vi "LiveAcquire Callback.vi"(4 "Config And DataQueues":T1 {"Config In"."Hardware Configuration"."Lasers Configuration"."SettingValues"."785 Power" format="%.1f"; "Config In"."Hardware Configuration"."Lasers Configuration"."SettingValues"."647 Power" format="%.1f"; "Config In"."Hardware Configuration"."Lasers Configuration"."SettingValues"."561 Power" format="%.1f"}, 5 "Event Data":cluster{"sender":refnum<k24>, "e":refnum<k24>}, 6 "Control Ref":refnum<k24>, 7 "Event Common Data":T10) -> ()   [LabVIEW 2019]
uses:
  C:/RM21-MMicrosopeSource/HardwareAdapter/Camera/Dependencies/PVCamNET.dll
  HardwareAdapter/Camera/Dependencies/PVCamNET.dll
  Config DataQueues And Notifier Ctl.ctl
  DataQueuesAndNotifier.ctl
  Settings/System Running Settings.ctl
  HardwareAdapter/Support/Hardware Configuration.ctl
  HardwareAdapter/Support/Camera Configuration.ctl
  <vilib>/vision/Image Controls.llb/IMAQ Image.ctl
  C:/RM21-MMicrosopeSource/HardwareAdapter/Lasers/Dependencies/Oxxius_Boxx.dll
  HardwareAdapter/Lasers/Dependencies/Oxxius_Boxx.dll
  Logging/Logging Configuration.ctl
  Controls/DeviceStatusCtl.ctl
  Controls/CallBack Refs.ctl
  Controls/Image MatadataCtl.ctl
  Global.vi
  Logging/Logging.lvlib
  Settings/Settings.lvlib
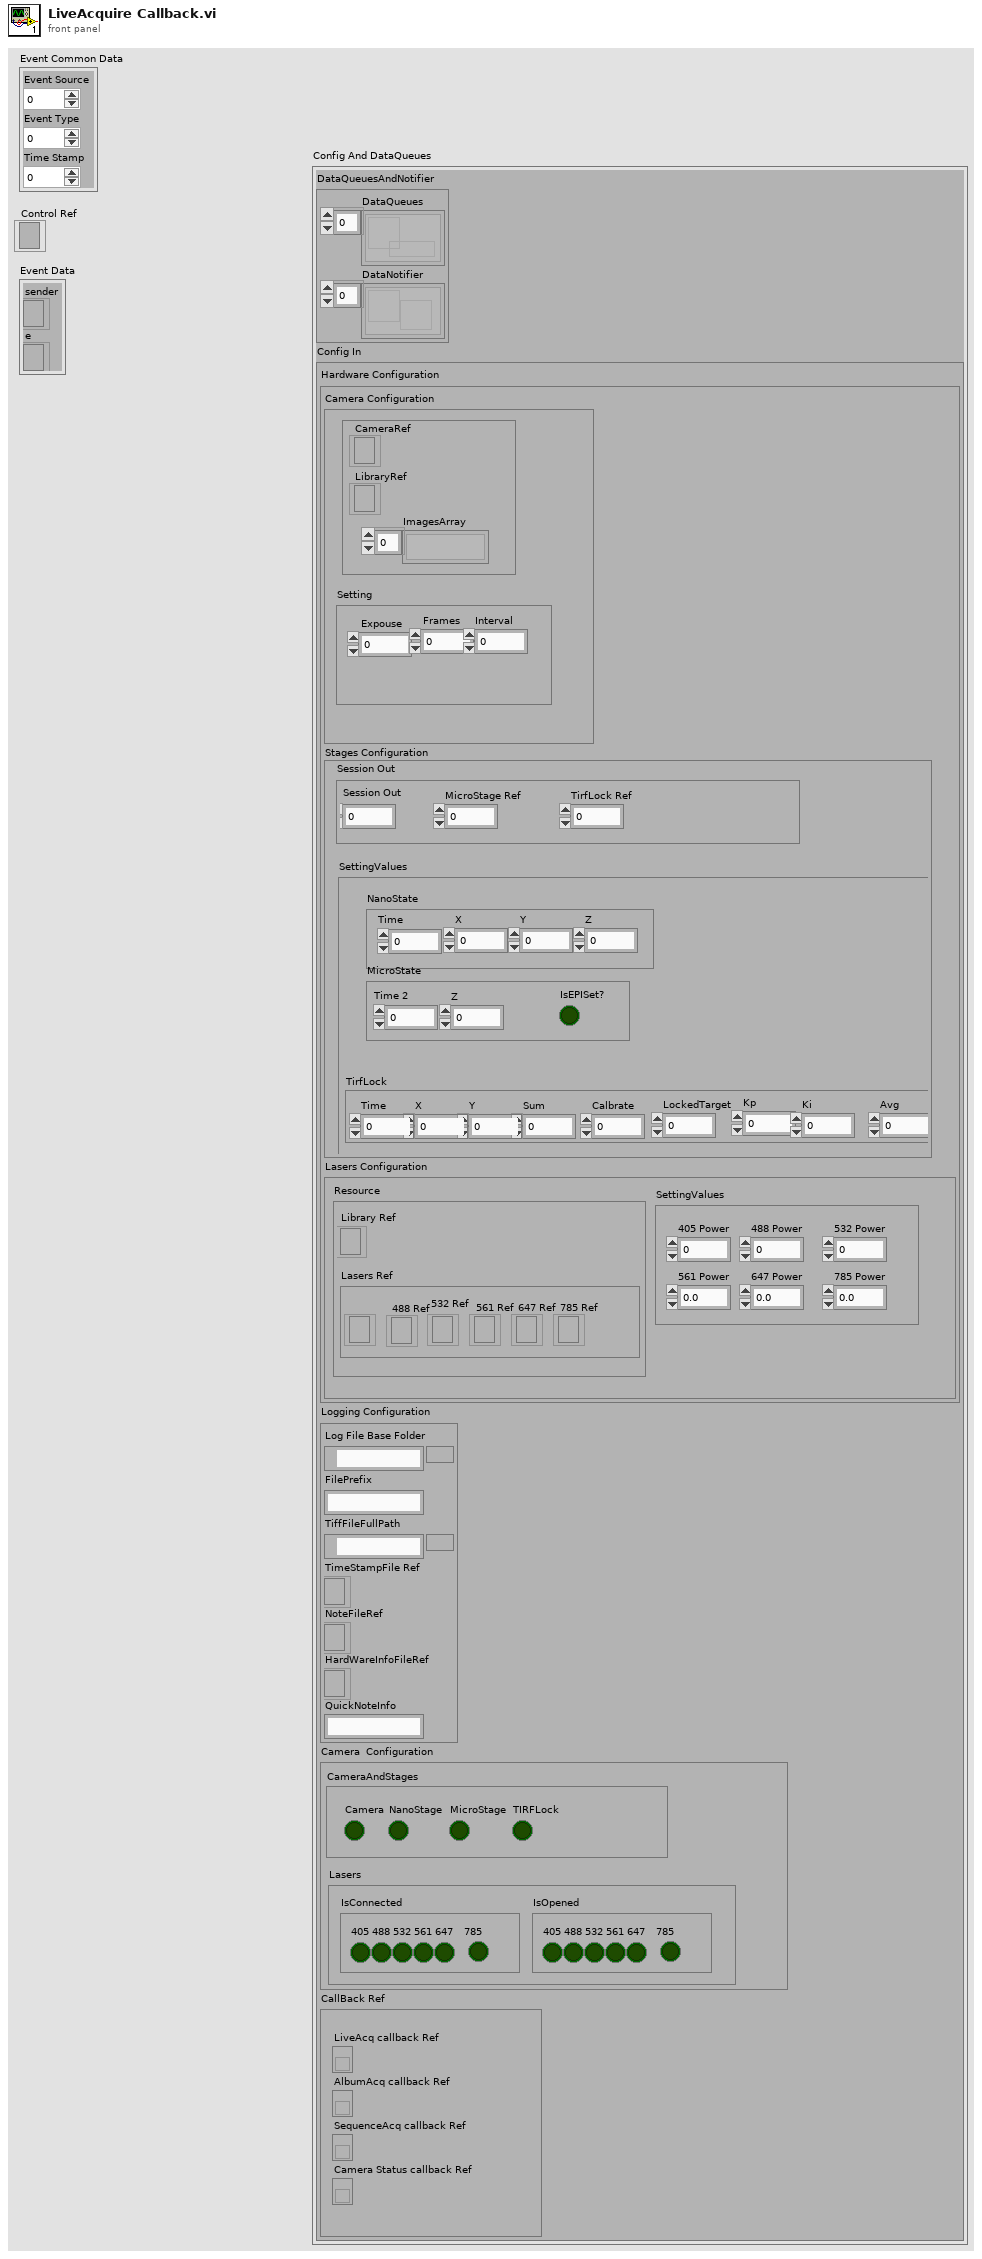
[diagram p1: front panel]
types:
  T1 = typedef "Config DataQueues And Notifier Ctl.ctl" = cluster{"DataQueuesAndNotifier":T2, "Config In":T3}
  T2 = typedef "DataQueuesAndNotifier.ctl" = cluster{"DataQueues":refnum<queue>[], "DataNotifier":refnum<notifier>[]}
  T3 = typedef "Settings.lvlib/System Running Settings.ctl" = cluster{"Hardware Configuration":T4, "Logging Configuration":T7, "HardWare Status":cluster{"CameraAndStages":T8, "Lasers":cluster{"IsConnected":cluster{"405":bool, "488":bool, "532":bool, "561":bool, "647":bool, "785":bool}, "IsOpened":cluster{"405":bool, "488":bool, "532":bool, "561":bool, "647":bool, "785":bool}}}, "CallBack Ref":T9}
  T4 = typedef "Hardware Configuration.ctl" = cluster{"Camera Configuration":T5, "Stages Configuration":cluster{"Resource":cluster{"NanoStage Ref":i32, "MicroStage Ref":i32, "TirfLock Ref":i32}, "SettingValues":cluster{"NanoState":cluster{"Time":dbl, "X":dbl, "Y":dbl, "Z":dbl}, "MicroState":cluster{"Time 2":dbl, "Z":dbl, "IsEPISet?":bool}, "TirfLock":cluster{"Time":dbl, "X":dbl, "Y":dbl, "Sum":dbl, "Calbrate":dbl, "LockedTarget":dbl, "Kp":dbl, "Ki":dbl, "Avg":dbl}}}, "Lasers Configuration":cluster{"SettingValues":cluster{"405 Power":sgl, "488 Power":sgl, "532 Power":sgl, "561 Power":sgl, "647 Power":sgl, "785 Power":sgl}, "Resource":cluster{"Library Ref":refnum<k24>, "Lasers Ref":cluster{"405 Ref":refnum<k24>, "488 Ref":refnum<k24>, "532 Ref":refnum<k24>, "561 Ref":refnum<k24>, "647 Ref":refnum<k24>, "785 Ref":refnum<k24>}}}}
  T5 = typedef "Camera Configuration.ctl" = cluster{"Setting":cluster{"Expouse":dbl, "Frames":dbl, "Interval":dbl}, "Resource":cluster{"CameraRef":refnum<k24>, "LibraryRef":refnum<k24>, "ImagesArray":T6[]}}
  T6 = typedef "IMAQ Image.ctl" = refnum<image>
  T7 = typedef "Logging.lvlib/Logging Configuration.ctl" = cluster{"Log File Base Folder":path, "FilePrefix":string, "TiffFileFullPath":path, "TimeStampFile Ref":refnum<file>, "NoteFileRef":refnum<file>, "HardWareInfoFileRef":refnum<file>, "QuickNoteInfo":string}
  T8 = typedef "DeviceStatusCtl.ctl" = cluster{"Camera":bool, "NanoStage":bool, "MicroStage":bool, "TIRFLock":bool}
  T9 = typedef "CallBack Refs.ctl" = cluster{"LiveAcq callback Ref":refnum<k27>, "AlbumAcq callback Ref":refnum<k27>, "SequenceAcq callback Ref":refnum<k27>, "Camera Status callback Ref":refnum<k27>}
  T10 = cluster{"Event Source":i32, "Event Type":u32, "Time Stamp":u32}
  T11 = typedef "Image MatadataCtl.ctl" = cluster{"EofTimeStamp(Acq)":dbl, "Image":T6, "Histogram":u32[], "MeanValue":dbl, "Min":u32, "Max":u32, "EofTimeStamp(Album)":dbl, "Fps":dbl, "BufferIndex":u32, "DroppedFrames":u32}
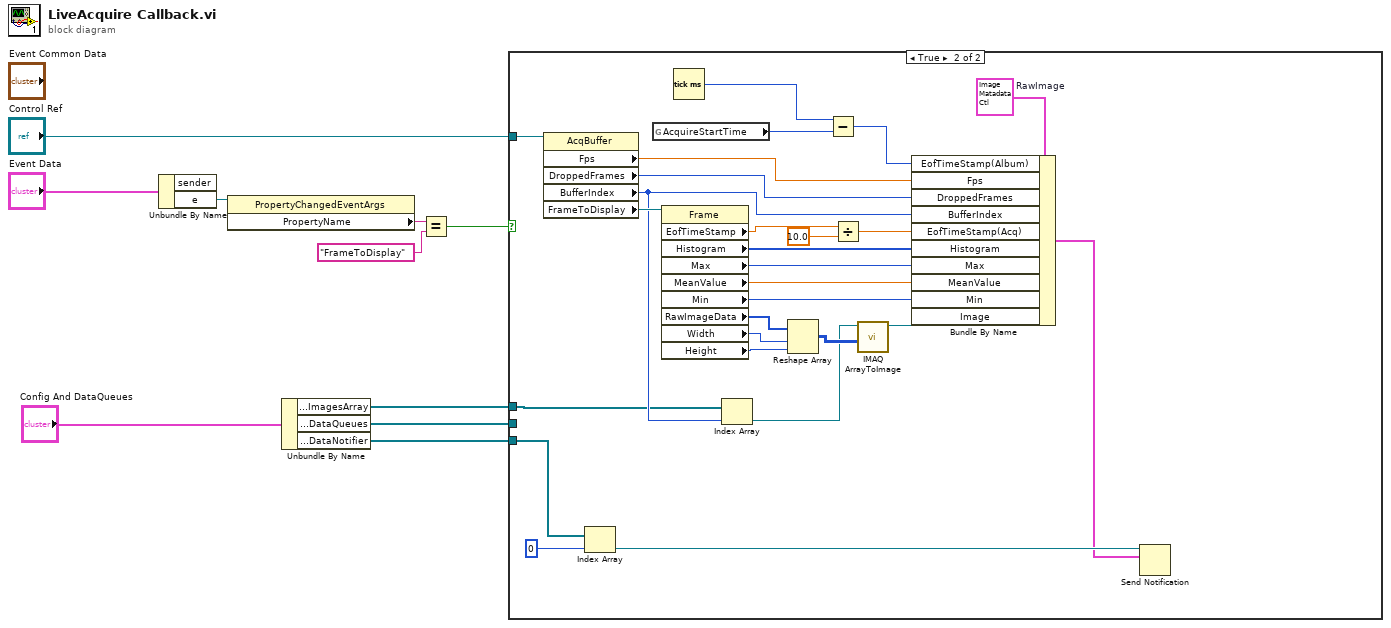
[diagram p0: block diagram]
diagram:
  n1 = Unbundle By Name("Event Data") -> ("e"=w9:refnum<k24>)  [unwired: 1 out]
  n2 = property class="PropertyChangedEventArgs"(reference=w9) -> ("PropertyName"=w8:string)  [unwired: 1 in, 2 out]
  n3 = Unbundle By Name("Config And DataQueues") -> ("Config In.Hardware Configuration.Camera Configuration.Resource.ImagesArray"=w3:T6[], "DataQueuesAndNotifier.DataQueues"=w2:refnum<queue>[], "DataQueuesAndNotifier.DataNotifier"=w1:refnum<notifier>[])
  n4 = Equal?(x=w8, y="FrameToDisplay") -> (x = y?=w6:bool)
  n5 = case shown="True" w6 {
    tunnel: "Control Ref" -> [_ w37]
    tunnel: w3 -> [_ w19]
    tunnel: w2 -> [_ _]
    tunnel: w1 -> [_ w17]
    frame False {
    }
    frame True {
      w26 = T11 {"EofTimeStamp(Acq)"=0.0, "Image"=refnum, "Histogram"=[], "MeanValue"=0.0, "Min"=0, "Max"=0, "EofTimeStamp(Album)"=0.0, "Fps"=0.0, "BufferIndex"=0, "DroppedFrames"=0}  # RawImage
      n6 = property class="AcqBuffer"(reference=w37) -> ("Fps"=w22:sgl, "DroppedFrames"=w21:i32, "BufferIndex"=w20:i32, "FrameToDisplay"=w36:refnum<k24>)  [unwired: 1 in, 2 out]
      n7 = Index Array(array=w17, index=0) -> (element=w15:refnum<notifier>)
      n8 = global read "Global.vi" "AcquireStartTime"() -> (w12:u32)
      n9 = property class="Frame"(reference=w36) -> ("EofTimeStamp"=w23:dbl, "Histogram"=w27:u32[], "Max"=w28:u32, "MeanValue"=w29:dbl, "Min"=w32:u32, "RawImageData"=w33:i16[], "Width"=w35:u32, "Height"=w34:u32)  [unwired: 1 in, 2 out]
      n10 = Tick Count (ms)() -> (millisecond timer value=w13:u32)
      n11 = Index Array(array=w19, index=w20) -> (element=w18:T6)
      n12 = Reshape Array "Reshape Array"(w33, w35, w34) -> (w31:i16[][])
      n13 = Subtract(x=w13, y=w12) -> (x-y=w11:u32)
      n14 = Divide(x=w23, y=10.0) -> (x/y=w24:dbl)
      n15 = call "IMAQ ArrayToImage"("Image Pixels (I16)"=w31, "Image"=w18) -> ("Image Out"=w30:T6)  [unwired: 8 in, 1 out]
      n16 = Bundle By Name(cluster=w26, "EofTimeStamp(Album)"=w11, "Fps"=w22, "DroppedFrames"=w21, "BufferIndex"=w20, "EofTimeStamp(Acq)"=w24, "Histogram"=w27, "Max"=w28, "MeanValue"=w29, "Min"=w32, "Image"=w30) -> (w14:T11)
      n17 = Send Notification(notification=w14, notifier=w15) -> ()  [unwired: 1 in, 2 out]
    }
  }
